vi "run_vi.vi"   [LabVIEW 2015]
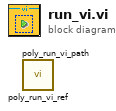
[diagram p0: block diagram]
diagram:
  n1 = call "poly_run_vi_ref.vi"() -> ()  [unwired: 7 in, 5 out]
  n2 = call "poly_run_vi_path.vi"() -> ()  [unwired: 7 in, 5 out]
